vi "Convert Num to Volts.vi"(1 "String":string) -> (0 "Numeric":dbl)   [LabVIEW 2013]
panel:
  out "Numeric (SI Notation)":dbl format="%#_6p"
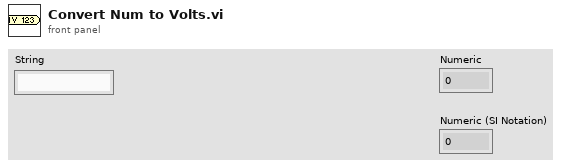
[diagram p1: front panel]
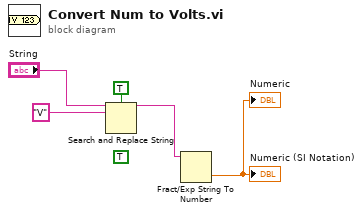
[diagram p0: block diagram]
diagram:
  (unwired) TRUE ("ignore case? (F)")
  n1 = Search and Replace String(case sensitive?=TRUE ("ignore case? (F)"), input string="String", search string="V") -> (result string=w2:string)  [unwired: 5 in, 3 out]
  n2 = Fract/Exp String To Number(string=w2) -> (number=→"Numeric" →"Numeric (SI Notation)":dbl)  [unwired: 3 in, 1 out]
